vi "U01_12UDPWrite.vi"() -> ()   [LabVIEW 2019]
panel:
  out "error out":errorcluster
  in  "error in (no error)":errorcluster
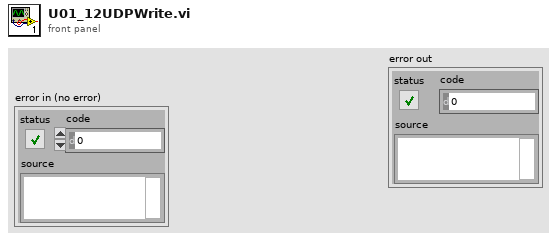
[diagram p1: front panel]
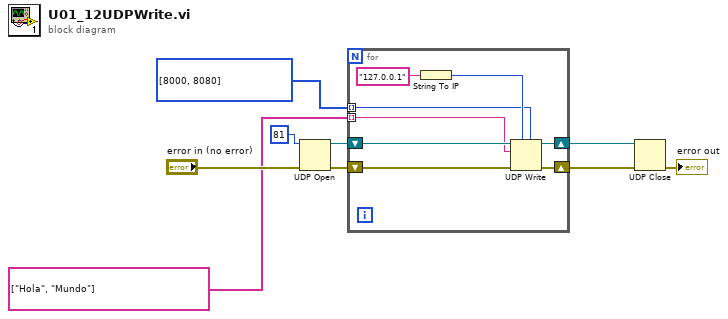
[diagram p0: block diagram]
diagram:
  n1 = UDP Open(8:"error in (no error)", 11:u16 81 ("port")) -> (port=w6:refnum<k16>, 0:w7:errorcluster)  [unwired: 3 in, 1 out]
  n2 = for {
    shift-right: [w12] -> w4
    shift-left: w7 -> [w17]
    shift-right: [w13] -> w5
    shift-left: w6 -> [w16]
    tunnel: string[] ["Hola", "Mundo"] -> [w11] mode=indexing
    tunnel: i32[] [8000, 8080] -> [w10] mode=indexing
    n3 = String To IP(1:"127.0.0.1") -> (0:w14:u32)
    n4 = UDP Write(address=w14, port or service name=w10, connection ID=w16, data in=w11, 8:w17) -> (error out=w12:errorcluster, 3:w13:refnum<k16>)  [unwired: 1 in]
  }
  n5 = UDP Close(connection ID=w5, 8:w4) -> (error out=→"error out":errorcluster)  [unwired: 1 out]
